vi "Overwrite Live Array at Specified Point.vi"(8 "error in (no error)":errorcluster, 9 "index":i32, 10 "New Processed Calibration Point":T2, 11 "Processed Calibration Points in":T1) -> (0 "error out":errorcluster, 3 "Processed Calibration Points out":T1)   [LabVIEW 2026, in "Processing_Engine.lvlib"]
uses:
  Processing_Engine.lvlib
  controls/Messaging Payloads/Processed Calibration Point.ctl
  controls/UI/Direction.ctl
  controls/Messaging Payloads/Processed Calibration Points.ctl
  Settings/Settings.lvlib
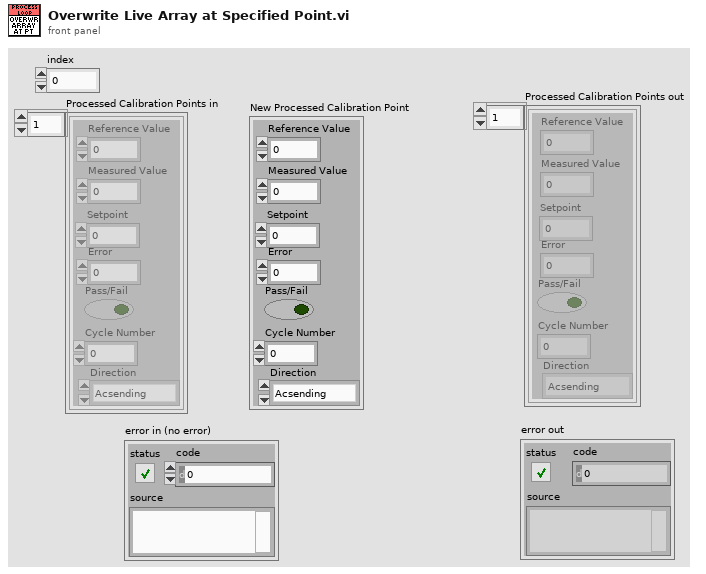
[diagram p1: front panel]
types:
  T1 = typedef "Processed Calibration Points.ctl" = T2[]
  T2 = typedef "Processed Calibration Point.ctl" = cluster{"Reference Value":dbl, "Measured Value":dbl, "Error":dbl, "Pass/Fail":bool, "Setpoint":dbl, "Cycle Number":i32, "Direction":T3}
  T3 = typedef "Settings.lvlib/Direction.ctl" = enum16{"Acsending", "Descending"}
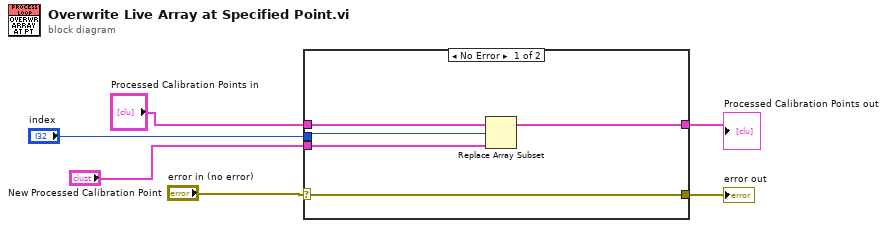
[diagram p0: block diagram]
diagram:
  n1 = case shown="No Error" "error in (no error)" {
    selector: "error in (no error)" -> [w8 w13]
    tunnel: "Processed Calibration Points in" -> [w11 w12]
    tunnel: "New Processed Calibration Point" -> [w7 _]
    tunnel: "index" -> [w10 _]
    tunnel: [w9 w12] -> w3
    tunnel: [w8 w13] -> w1
    frame No Error {
      n2 = Replace Array Subset(array=w11, new element=w7, index=w10) -> (w9:T1)
    }
    frame Error {
    }
  }
  "error out" <- w1
  "Processed Calibration Points out" <- w3
